vi "Calculate Rows To Draw.vi"(0 "reference in":refnum<class "Manipulator.lvclass">, 5 "WhichAxis?":string="x", 7 "InData":T2, 11 "error in (no error)":errorcluster) -> (3 "ArrayOfAngles":T1(array[cluster]), 4 "reference out":refnum<class "Manipulator.lvclass">, 6 "X":dbl[][](array[numeric]), 8 "Y":dbl[][](array[numeric]), 10 "Z":dbl[][](array[numeric]), 15 "error out":errorcluster)   [LabVIEW 2014, in "Manipulator.lvclass"]
uses:
  Manipulator.lvclass
  typedefs/Coordinates.ctl
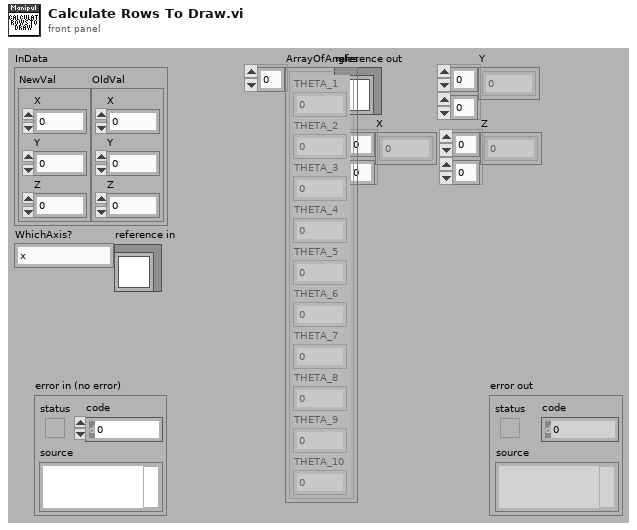
[diagram p1: front panel]
types:
  T1 = cluster{"THETA_1":dbl, "THETA_2":dbl, "THETA_3":dbl, "THETA_4":dbl, "THETA_5":dbl, "THETA_6":dbl, "THETA_7":dbl, "THETA_8":dbl, "THETA_9":dbl, "THETA_10":dbl}[]
  T2 = cluster{"NewVal":cluster{"X":dbl, "Y":dbl, "Z":dbl}, "OldVal":cluster{"X":dbl, "Y":dbl, "Z":dbl}}
  T3 = typedef "Manipulator.lvclass/Coordinates.ctl" = cluster{"X":dbl, "Y":dbl, "Z":dbl}
  T4 = cluster{"THETA_1":dbl, "THETA_2":dbl, "THETA_3":dbl, "THETA_4":dbl, "THETA_5":dbl, "THETA_6":dbl, "THETA_7":dbl, "THETA_8":dbl, "THETA_9":dbl, "THETA_10":dbl}
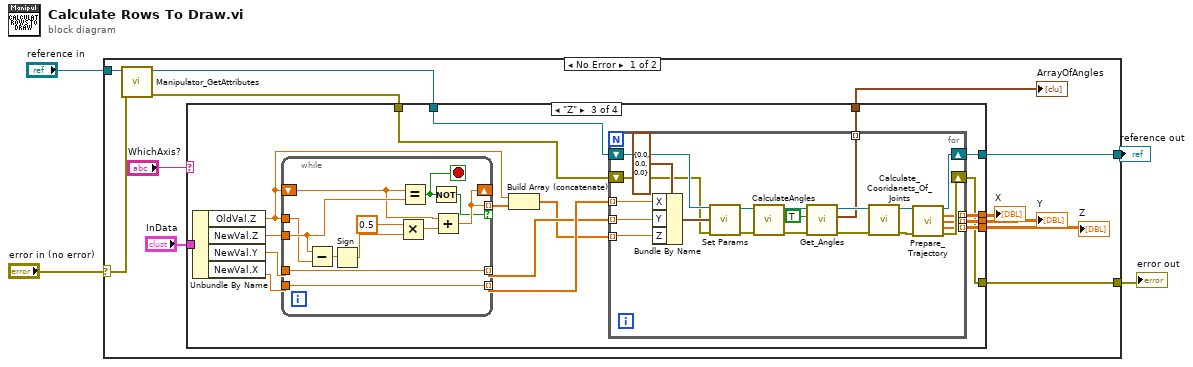
[diagram p0: block diagram]
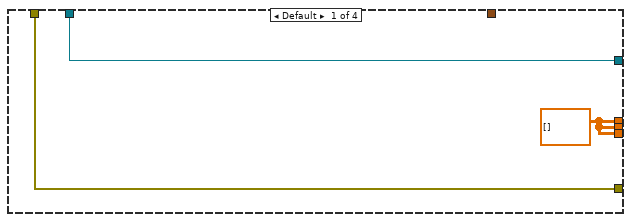
[diagram p2: hidden frame]
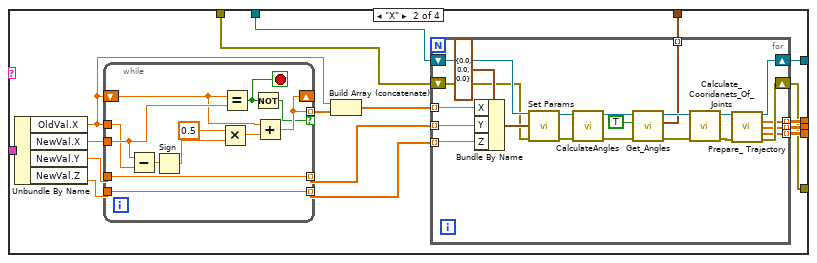
[diagram p3: hidden frame]
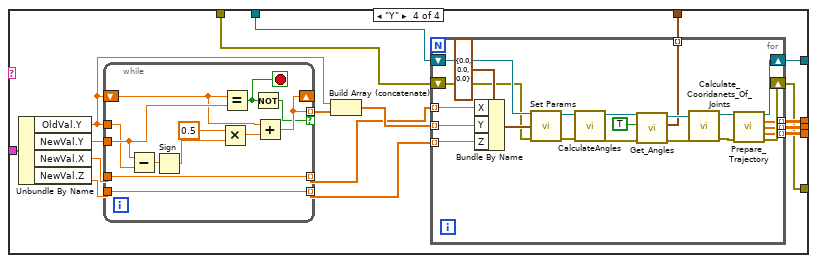
[diagram p4: hidden frame]
diagram:
  n1 = case shown="No Error" "error in (no error)" {
    selector: "error in (no error)" -> [w13 w174]
    tunnel: [w6 w174] -> w3
    tunnel: "reference in" -> [w14 w173]
    tunnel: [w10 w173] -> w1
    frame No Error {
      n2 = call "Manipulator_GetAttributes.vi"("error in (no error)"=w13, "reference in"=w14) -> ("error out"=w11:errorcluster, "reference out"=w12:refnum<class "Manipulator.lvclass">)  [unwired: 6 in, 2 out]
      n3 = case shown="\"Z\"" "WhichAxis?" {
        tunnel: "InData" -> [_ w28 w82 w132]
        tunnel: w12 -> [w19 w26 w80 w130]
        tunnel: w11 -> [w18 w27 w81 w131]
        tunnel: [w19 w25 w79 w129] -> w10
        tunnel: [w17 w24 w78 w128] -> w9
        tunnel: [w17 w23 w77 w127] -> w8
        tunnel: [w17 w22 w76 w126] -> w7
        tunnel: [w18 w21 w75 w125] -> w6
        tunnel: [_ w20 w71 w122] -> w5
        frame Default {
          w17 = dbl[][] [] ("X")
        }
        frame "X" {
          n4 = Unbundle By Name(w28) -> ("OldVal.X"=w34:dbl, "NewVal.X"=w36:dbl, "NewVal.Y"=w33:dbl, "NewVal.Z"=w32:dbl)
          n5 = while {
            tunnel: w34 -> [w69]
            tunnel: w36 -> [w70]
            shift-right: [w64] -> _
            shift-left: w34 -> [w63]
            tunnel: [w64] -> w35 mode=indexing if=w61
            tunnel: w33 -> [w60]
            tunnel: w32 -> [w59]
            tunnel: [w60] -> w30 mode=indexing
            tunnel: [w59] -> w29 mode=indexing
            stop <- w62 stop-if-true
            n6 = Subtract(x=w70, y=w69) -> (x-y=w68:dbl)
            n7 = Sign(1:w68) -> (0:w66:dbl)
            n8 = Multiply(x=0.5 ("y"), y=w66) -> (x*y=w67:dbl)
            n9 = Equal?(x=w63, y=w70) -> (x = y?=w62:bool)
            n10 = Not(x=w62) -> (.not. x?=w61:bool)
            n11 = Add(x=w63, y=w67) -> (x+y=w64:dbl)
          }
          n12 = Build Array (concatenate)(w34, w35) -> (w31:dbl[])
          n13 = for {
            shift-right: [w46] -> w21
            shift-left: w27 -> [w50]
            shift-right: [w47] -> w25
            shift-left: w26 -> [w51]
            tunnel: w31 -> [w55] mode=indexing
            tunnel: w30 -> [w54] mode=indexing
            tunnel: w29 -> [w53] mode=indexing
            tunnel: [w45] -> w24 mode=indexing
            tunnel: [w44] -> w23 mode=indexing
            tunnel: [w43] -> w22 mode=indexing
            tunnel: [w38] -> w20 mode=indexing
            n14 = Bundle By Name(cluster=T3 {"X"=0.0, "Y"=0.0, "Z"=0.0} ("CoordinatesIN"), "X"=w55, "Y"=w54, "Z"=w53) -> (w58:T3)
            n15 = call-dynamic "Set Params.vi"("error in (no error)"=w50, "CoordinatesIN"=w58, "reference in"=w51) -> ("error out"=w57:errorcluster, "reference out"=w56:refnum<class "Manipulator.lvclass">)  [unwired: 7 in]
            n16 = call "CalculateAngles.vi"("error in (no error)"=w57, "reference in"=w56) -> ("error out"=w39:errorcluster, "reference out"=w40:refnum<class "Manipulator.lvclass">)  [unwired: 8 in]
            n17 = call-dynamic "Get_Angles.vi"("error in (no error)"=w39, "Deg?"=TRUE, "reference in"=w40) -> ("error out"=w42:errorcluster, "Angles"=w38:T4, "reference out"=w41:refnum<class "Manipulator.lvclass">)  [unwired: 6 in]
            n18 = call-dynamic "Calculate_Cooridanets_Of_Joints.vi"("error in (no error)"=w42, "reference in"=w41) -> ("error out"=w48:errorcluster, "reference out"=w49:refnum<class "Manipulator.lvclass">)  [unwired: 8 in]
            n19 = call-dynamic "Prepare_ Trajectory.vi"("reference in"=w49, "error in (no error)"=w48) -> ("reference out"=w47:refnum<class "Manipulator.lvclass">, "X"=w45:dbl[], "Y"=w44:dbl[], "Z"=w43:dbl[], "error out"=w46:errorcluster)  [unwired: 9 in]
          }
        }
        frame "Z" {
          n20 = Unbundle By Name(w82) -> ("OldVal.Z"=w85:dbl, "NewVal.Z"=w87:dbl, "NewVal.Y"=w84:dbl, "NewVal.X"=w83:dbl)
          n21 = while {
            tunnel: w85 -> [w120]
            tunnel: w87 -> [w121]
            shift-right: [w115] -> _
            shift-left: w85 -> [w114]
            tunnel: [w115] -> w86 mode=indexing if=w112
            tunnel: w84 -> [w111]
            tunnel: w83 -> [w110]
            tunnel: [w111] -> w73 mode=indexing
            tunnel: [w110] -> w74 mode=indexing
            stop <- w113 stop-if-true
            n22 = Subtract(x=w121, y=w120) -> (x-y=w119:dbl)
            n23 = Sign(1:w119) -> (0:w117:dbl)
            n24 = Multiply(x=0.5 ("y"), y=w117) -> (x*y=w118:dbl)
            n25 = Equal?(x=w114, y=w121) -> (x = y?=w113:bool)
            n26 = Not(x=w113) -> (.not. x?=w112:bool)
            n27 = Add(x=w114, y=w118) -> (x+y=w115:dbl)
          }
          n28 = Build Array (concatenate)(w85, w86) -> (w72:dbl[])
          n29 = for {
            shift-right: [w97] -> w75
            shift-left: w81 -> [w101]
            shift-right: [w98] -> w79
            shift-left: w80 -> [w102]
            tunnel: w74 -> [w106] mode=indexing
            tunnel: w73 -> [w105] mode=indexing
            tunnel: w72 -> [w104] mode=indexing
            tunnel: [w96] -> w78 mode=indexing
            tunnel: [w95] -> w77 mode=indexing
            tunnel: [w94] -> w76 mode=indexing
            tunnel: [w89] -> w71 mode=indexing
            n30 = Bundle By Name(cluster=T3 {"X"=0.0, "Y"=0.0, "Z"=0.0} ("CoordinatesIN"), "X"=w106, "Y"=w105, "Z"=w104) -> (w109:T3)
            n31 = call-dynamic "Set Params.vi"("error in (no error)"=w101, "CoordinatesIN"=w109, "reference in"=w102) -> ("error out"=w108:errorcluster, "reference out"=w107:refnum<class "Manipulator.lvclass">)  [unwired: 7 in]
            n32 = call "CalculateAngles.vi"("error in (no error)"=w108, "reference in"=w107) -> ("error out"=w93:errorcluster, "reference out"=w92:refnum<class "Manipulator.lvclass">)  [unwired: 8 in]
            n33 = call-dynamic "Get_Angles.vi"("error in (no error)"=w93, "Deg?"=TRUE, "reference in"=w92) -> ("error out"=w90:errorcluster, "Angles"=w89:T4, "reference out"=w91:refnum<class "Manipulator.lvclass">)  [unwired: 6 in]
            n34 = call-dynamic "Calculate_Cooridanets_Of_Joints.vi"("error in (no error)"=w90, "reference in"=w91) -> ("error out"=w99:errorcluster, "reference out"=w100:refnum<class "Manipulator.lvclass">)  [unwired: 8 in]
            n35 = call-dynamic "Prepare_ Trajectory.vi"("reference in"=w100, "error in (no error)"=w99) -> ("reference out"=w98:refnum<class "Manipulator.lvclass">, "X"=w96:dbl[], "Y"=w95:dbl[], "Z"=w94:dbl[], "error out"=w97:errorcluster)  [unwired: 9 in]
          }
        }
        frame "Y" {
          n36 = Unbundle By Name(w132) -> ("OldVal.Y"=w136:dbl, "NewVal.Y"=w138:dbl, "NewVal.X"=w135:dbl, "NewVal.Z"=w134:dbl)
          n37 = while {
            tunnel: w136 -> [w171]
            tunnel: w138 -> [w172]
            shift-right: [w166] -> _
            shift-left: w136 -> [w165]
            tunnel: [w166] -> w137 mode=indexing if=w163
            tunnel: w135 -> [w162]
            tunnel: w134 -> [w161]
            tunnel: [w162] -> w123 mode=indexing
            tunnel: [w161] -> w133 mode=indexing
            stop <- w164 stop-if-true
            n38 = Subtract(x=w172, y=w171) -> (x-y=w170:dbl)
            n39 = Sign(1:w170) -> (0:w168:dbl)
            n40 = Multiply(x=0.5 ("y"), y=w168) -> (x*y=w169:dbl)
            n41 = Equal?(x=w165, y=w172) -> (x = y?=w164:bool)
            n42 = Not(x=w164) -> (.not. x?=w163:bool)
            n43 = Add(x=w165, y=w169) -> (x+y=w166:dbl)
          }
          n44 = Build Array (concatenate)(w136, w137) -> (w124:dbl[])
          n45 = for {
            shift-right: [w148] -> w125
            shift-left: w131 -> [w152]
            shift-right: [w149] -> w129
            shift-left: w130 -> [w153]
            tunnel: w123 -> [w157] mode=indexing
            tunnel: w124 -> [w156] mode=indexing
            tunnel: w133 -> [w155] mode=indexing
            tunnel: [w147] -> w128 mode=indexing
            tunnel: [w146] -> w127 mode=indexing
            tunnel: [w145] -> w126 mode=indexing
            tunnel: [w139] -> w122 mode=indexing
            n46 = Bundle By Name(cluster=T3 {"X"=0.0, "Y"=0.0, "Z"=0.0} ("CoordinatesIN"), "X"=w157, "Y"=w156, "Z"=w155) -> (w160:T3)
            n47 = call-dynamic "Set Params.vi"("error in (no error)"=w152, "CoordinatesIN"=w160, "reference in"=w153) -> ("error out"=w159:errorcluster, "reference out"=w158:refnum<class "Manipulator.lvclass">)  [unwired: 7 in]
            n48 = call "CalculateAngles.vi"("error in (no error)"=w159, "reference in"=w158) -> ("error out"=w144:errorcluster, "reference out"=w143:refnum<class "Manipulator.lvclass">)  [unwired: 8 in]
            n49 = call-dynamic "Get_Angles.vi"("error in (no error)"=w144, "Deg?"=TRUE, "reference in"=w143) -> ("error out"=w140:errorcluster, "Angles"=w139:T4, "reference out"=w141:refnum<class "Manipulator.lvclass">)  [unwired: 6 in]
            n50 = call-dynamic "Calculate_Cooridanets_Of_Joints.vi"("error in (no error)"=w140, "reference in"=w141) -> ("error out"=w150:errorcluster, "reference out"=w151:refnum<class "Manipulator.lvclass">)  [unwired: 8 in]
            n51 = call-dynamic "Prepare_ Trajectory.vi"("reference in"=w151, "error in (no error)"=w150) -> ("reference out"=w149:refnum<class "Manipulator.lvclass">, "X"=w147:dbl[], "Y"=w146:dbl[], "Z"=w145:dbl[], "error out"=w148:errorcluster)  [unwired: 9 in]
          }
        }
      }
      "X" <- w9
      "Y" <- w8
      "Z" <- w7
      "ArrayOfAngles" <- w5
    }
    frame Error {
    }
  }
  "error out" <- w3
  "reference out" <- w1
